vi "ConnStrToParams.vi"(8 "error in (no error)":errorcluster, 10 "Connection String":string, 11 "CameraDemo in":refnum<class "Camera.lvclass">) -> (0 "error out":errorcluster, 3 "CameraDemo out":refnum<class "Camera.lvclass">)   [LabVIEW 2020, in "CameraI2COUSB.lvlib" / "Camera.lvclass"]
uses:
  Camera.lvclass
  Camera.lvclass/Camera.ctl
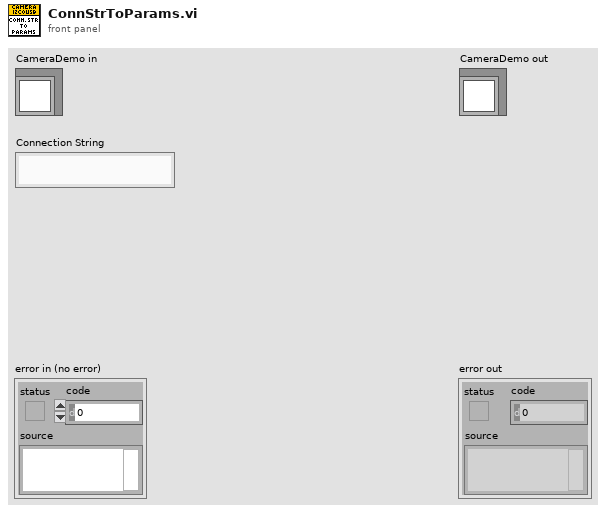
[diagram p1: front panel]
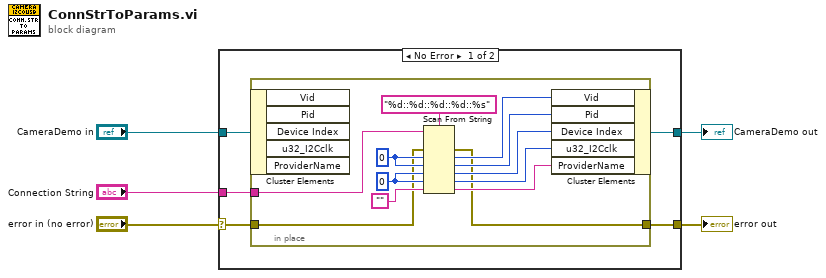
[diagram p0: block diagram]
diagram:
  n1 = case shown="No Error" "error in (no error)" {
    selector: "error in (no error)" -> [w8 w24]
    tunnel: [w7 w24] -> w4
    tunnel: [w9 w23] -> w2
    tunnel: "CameraDemo in" -> [w10 w23]
    tunnel: "Connection String" -> [w6 _]
    frame No Error {
      n2 = in-place {
        in-place-border: w8 -> [w13]
        in-place-border: [w12] -> w7
        in-place-border: w6 -> [w11]
        w20 = u32 0
        w21 = u16 0
        n3 = in-place-cluster #1(w10) -> ()  [unwired: 5 out]
        n4 = Scan From String(format string="%d::%d::%d::%d::%s", input string=w11, error in=w13, default 1=w21, default 2=w21, default 3=w20, default 4=w20, default 5="") -> (error out=w12:errorcluster, output 1=w18:u16, output 2=w17:u16, output 3=w16:u32, output 4=w15:u32, output 5=w14:string)  [unwired: 1 in, 2 out]
        n5 = in-place-cluster #1("Vid"=w18, "Pid"=w17, "Device Index"=w16, "u32_I2Cclk"=w15, "ProviderName"=w14) -> (w9:refnum<class "Camera.lvclass">)
      }
    }
    frame Error {
    }
  }
  "error out" <- w4
  "CameraDemo out" <- w2
